vi "String Get String.vi"(8 "error in (no error)":errorcluster, 11 "String DVR in":refnum<data-value>) -> (0 "error out":errorcluster, 2 "String value out":string, 3 "String DVR out":refnum<data-value>)   [LabVIEW 2010, in "MDSplus.lvlib"]
uses:
  <vilib>/MDSplus/Library/MDSplus.lvlib
  <vilib>/MDSplus/Classes/Data_Class/Scalar_Class/String_Class/String.lvclass
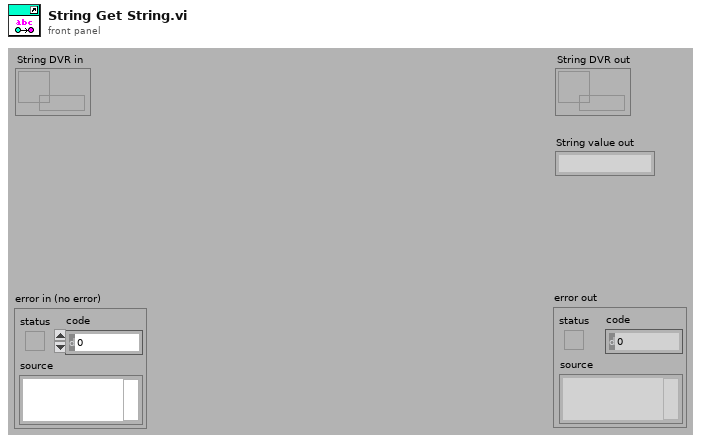
[diagram p1: front panel]
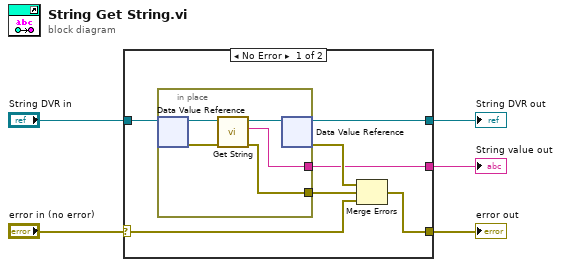
[diagram p0: block diagram]
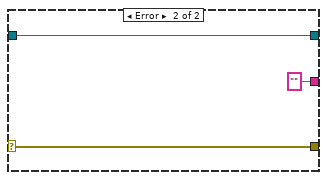
[diagram p2: hidden frame]
diagram:
  n1 = case shown="No Error" "error in (no error)" {
    selector: "error in (no error)" -> [w10 w20]
    tunnel: "String DVR in" -> [w12 w19]
    tunnel: [w8 w20] -> w5
    tunnel: [w7 w19] -> w1
    tunnel: [w6 "" ("String value out")] -> w4
    frame No Error {
      n2 = in-place {
        in-place-border: [w15] -> w11
        in-place-border: [w13] -> w6
        n3 = in-place-dvr #1(w12) -> (w17:refnum<class "String.lvclass">, w14:errorcluster)
        n4 = call-dynamic "Get String.vi"("error in (no error)"=w14, "String in"=w17) -> ("error out"=w15:errorcluster, "String value out"=w13:string, "String out"=w16:refnum<class "String.lvclass">)  [unwired: 7 in]
        n5 = in-place-dvr #1(w16) -> (w7:refnum<data-value>, w9:errorcluster)
      }
      n6 = Merge Errors(w9, w11, w10) -> (w8:errorcluster)
    }
    frame Error {
    }
  }
  "error out" <- w5
  "String value out" <- w4
  "String DVR out" <- w1
